vi "solar_voy Release.vi"(6 "Suppress Errors? (T)":bool=TRUE, 8 "error in (no error)":errorcluster, 10 "Force Destroy? (F)":bool, 11 "Voyager Refnum":T10) -> (0 "error out":errorcluster, 3 "Voyager":T1 {"PACKETS"."last_time" format="%<%H:%M:%S%3u %m/%d/%y>T"})   [LabVIEW 2018]
doc: "This releases the Voyager reference. Set <b>Force Destroy?</b> to true, to destroy the reference."
uses:
  solar_voy_ctl Voyager Refnum.ctl
  solar_voy_ctl Voyager.ctl
  solar_voy_def/solar_voy_def_ctl ITEM TYPE.ctl
  type/solar_type Item Type.ctl
  solar_voy_def/solar_voy_def_ctl ITEM.ctl
  solar_voy_def/solar_voy_def_ctl PACKET.ctl
  solar_voy_def/solar_voy_def_ctl PACKET_ID.ctl
  solar_voy_def/solar_voy_def_ctl HDR.ctl
  solar_voy_ctl TCP.ctl
  solar_voy_ctl Port Setup.ctl
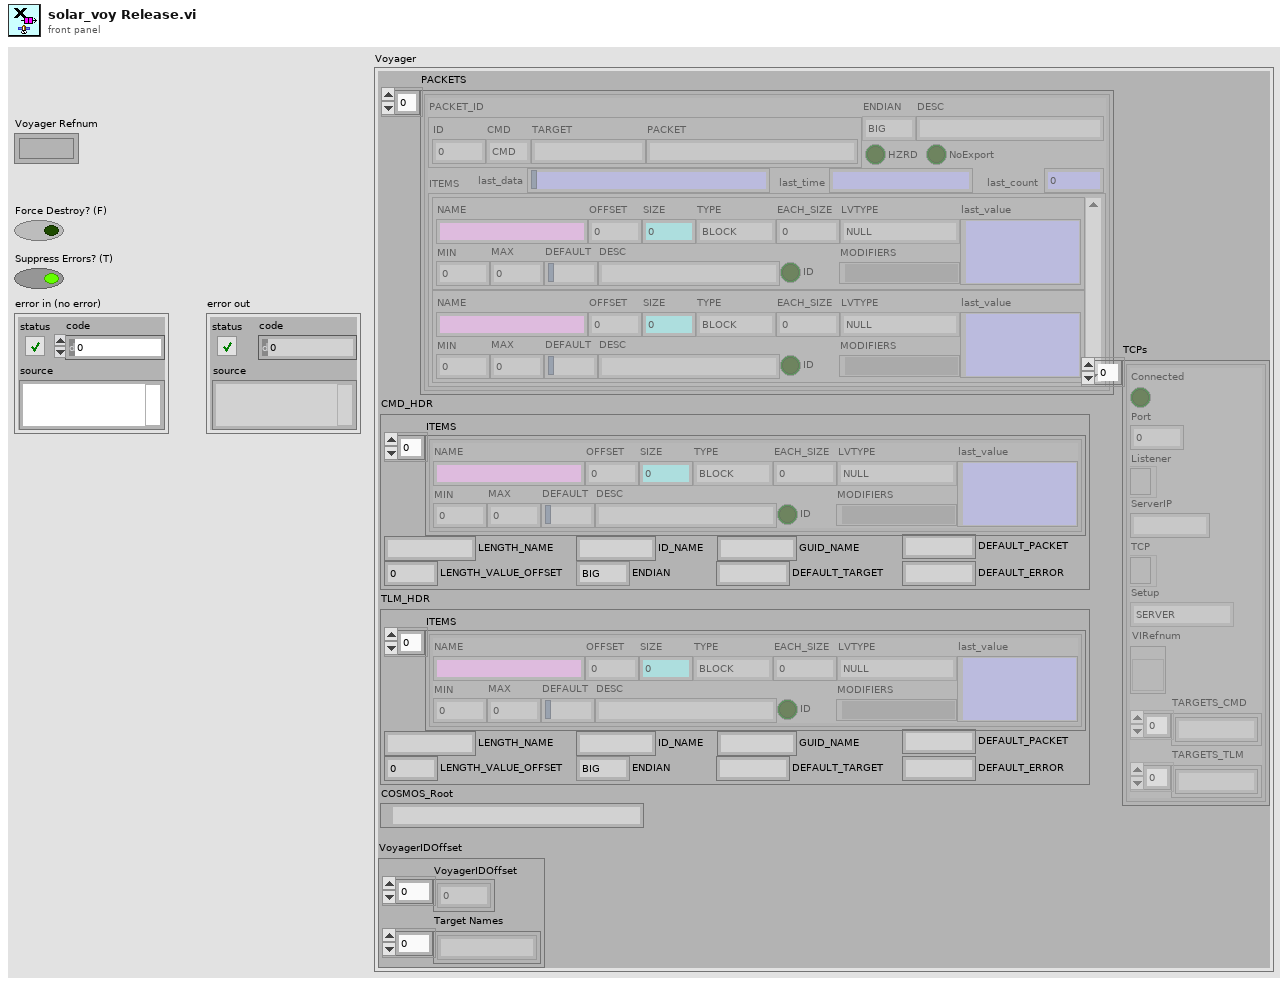
[diagram p1: front panel]
types:
  T1 = typedef "solar_voy_ctl Voyager.ctl" = cluster{"PACKETS":T2[], "COSMOS_Root":path, "CMD_HDR":T7, "TLM_HDR":T7, "TCPs":T8[], "VoyagerIDOffset":cluster{"VoyagerIDOffset":u16[], "Target Names":string[]}}
  T2 = typedef "solar_voy_def_ctl PACKET.ctl" = cluster{"PACKET_ID":T3, "ENDIAN":enum8{"BIG", "LITTLE"}, "DESC":string, "HZRD":bool, "ITEMS":T4[], "NoExport":bool, "last_time":timestamp, "last_count":u32, "last_data":string}
  T3 = typedef "solar_voy_def_ctl PACKET_ID.ctl" = cluster{"ID":u16, "CMD":enum8{"CMD", "TLM"}, "TARGET":string, "PACKET":string}
  T4 = typedef "solar_voy_def_ctl ITEM.ctl" = cluster{"NAME":string, "OFFSET":i32, "SIZE":i32, "TYPE":T5, "EACH_SIZE":i32, "LVTYPE":T6, "MIN":dbl, "MAX":dbl, "DEFAULT":string, "DESC":string, "ID":bool, "MODIFIERS":variant, "last_value":variant}
  T5 = typedef "solar_voy_def_ctl ITEM TYPE.ctl" = enum8{"BLOCK", "INT", "UINT", "FLOAT", "STRING"}
  T6 = typedef "solar_type Item Type.ctl" = enum16{"NULL", "UNKNOWN", "CLUSTER", "I8", "I16", "I32", "I64", "U8", "U16", "U32", "U64", "U8_ENUM", "U16_ENUM", "U32_ENUM", "SGL", "DBL", "BOOLEAN", "STRING", "PATH", "VISA", "TAG", "TIME", "I8_1D", "I16_1D", "I32_1D", "I64_1D", "U8_1D", "U16_1D", "U32_1D", "U64_1D", "U8_ENUM_1D", "U16_ENUM_1D", "U32_ENUM_1D", "SGL_1D", "DBL_1D", "BOOLEAN_1D", "STRING_1D", "PATH_1D", "VISA_1D", "TAG_1D", "TIME_1D", "I8_2D", "I16_2D", "I32_2D", "I64_2D", "U8_2D", "U16_2D", "U32_2D", "U64_2D", "U8_ENUM_2D", "U16_ENUM_2D", "U32_ENUM_2D", "SGL_2D", "DBL_2D", "BOOLEAN_2D", "STRING_2D", "PATH_2D", "VISA_2D", "TAG_2D", "TIME_2D"}
  T7 = typedef "solar_voy_def_ctl HDR.ctl" = cluster{"ITEMS":T4[], "LENGTH_NAME":string, "LENGTH_VALUE_OFFSET":i32, "ID_NAME":string, "ENDIAN":enum8{"BIG", "LITTLE"}, "GUID_NAME":string, "DEFAULT_TARGET":string, "DEFAULT_PACKET":string, "DEFAULT_ERROR":string}
  T8 = typedef "solar_voy_ctl TCP.ctl" = cluster{"Connected":bool, "Port":u16, "Listener":refnum<k5>, "ServerIP":string, "TCP":refnum<k5>, "Setup":T9, "VIRefnum":refnum<vi>, "TARGETS_CMD":string[], "TARGETS_TLM":string[]}
  T9 = typedef "solar_voy_ctl Port Setup.ctl" = enum8{"SERVER", "CLIENT", "SERVER_CMD", "SERVER_TLM"}
  T10 = typedef "solar_voy_ctl Voyager Refnum.ctl" = refnum<k1>
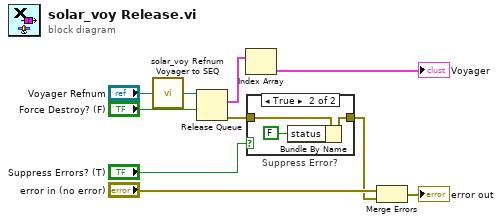
[diagram p0: block diagram]
diagram:
  n1 = call "solar_voy Refnum Voyager to SEQ.vi"("Voyager Refnum"="Voyager Refnum") -> ("Voyager SEQ"=w5:refnum<queue>)
  n2 = Release Queue(queue=w5, force destroy? (F)="Force Destroy? (F)") -> (remaining elements=w4:T1[], error out=w1:errorcluster)  [unwired: 1 in, 1 out]
  n3 = Index Array(array=w4) -> (element=→"Voyager":T1)  [unwired: 1 in]
  n4 = case "Suppress Error?" shown="True" "Suppress Errors? (T)" {
    tunnel: w1 -> [w11 w14]
    tunnel: [w11 w13] -> w8
    frame False {
    }
    frame True {
      n5 = Bundle By Name(cluster=w14, "status"=FALSE) -> (w13:errorcluster)
    }
  }
  n6 = Merge Errors("error in (no error)", w8) -> (→"error out":errorcluster)
